vi "Config Hash.vi"(8 "error in (no error)":errorcluster, 11 "VolatusAPI in":refnum<class "VolatusAPI.lvclass">) -> (0 "error out":errorcluster, 2 "Config Hash":string, 3 "VolatusAPI out":refnum<class "VolatusAPI.lvclass">)   [LabVIEW 2020, in "Volatus.lvlib" / "VolatusAPI.lvclass"]
uses:
  VolatusAPI.lvclass
  VolatusAPI.lvclass/VolatusAPI.ctl
  VolatusConfig/VolatusConfig/VolatusConfig.lvclass
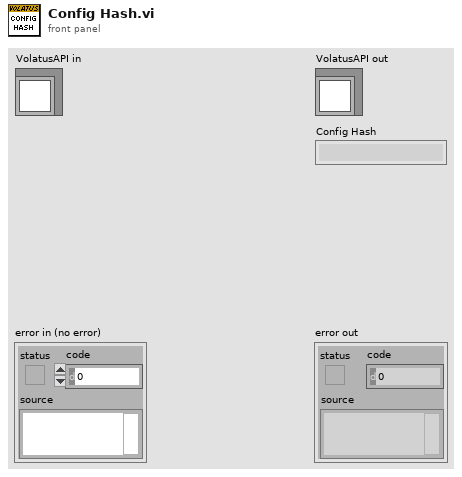
[diagram p1: front panel]
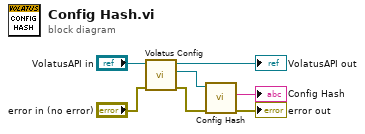
[diagram p0: block diagram]
diagram:
  n1 = call "Volatus Config.vi"("error in (no error)"="error in (no error)", "VolatusAPI in"="VolatusAPI in") -> ("error out"=w3:errorcluster, "Volatus Config"=w5:refnum<class "VolatusConfig.lvclass">, "VolatusAPI out"=→"VolatusAPI out":refnum<class "VolatusAPI.lvclass">)  [unwired: 7 in]
  n2 = call "Config Hash.vi"("error in (no error)"=w3, "VolatusConfig in"=w5) -> ("error out"=→"error out":errorcluster, "Config Hash"=→"Config Hash":string)  [unwired: 7 in, 1 out]
